vi "Public Application Data Folder.vi"(3 "Relative Path (\"\" - Folder)":string) -> (1 "Client Storage Path":path)   [LabVIEW 2011]
uses:
  <vilib>/Utility/sysdir.llb/System Directory Type.ctl
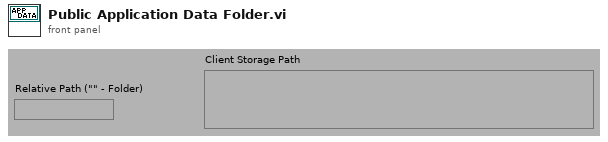
[diagram p1: front panel]
types:
  T1 = enum32{"invalid app kind", "Development System", "Run Time System", "Student Edition", "Embedded LabVIEW", "Evaluation", "Custom"}
  T2 = typedef "System Directory Type.ctl" = i32
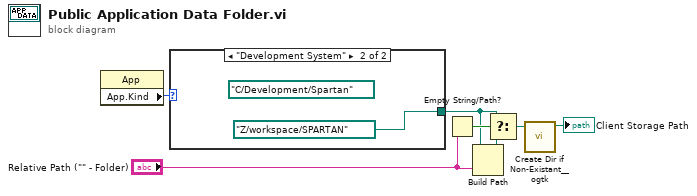
[diagram p0: block diagram]
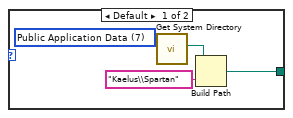
[diagram p2: hidden frame]
diagram:
  n1 = property class="App"() -> ("App.Kind"=w7:T1)  [unwired: 2 in, 2 out]
  n2 = case shown="\"Development System\"" w7 {
    tunnel: [w8 path "Z:/workspace/SPARTAN" ("appended path")] -> w3
    frame Default {
      w10 = T2 7 items=["User Home", "User Desktop", "User Documents", "User Application Data", "User Preferences", "User Temporary", "Public Documents", "Public Application Data", "Public Preferences", "System Core Libraries", "System Installed Libraries", "Application Files", "Boot Volume Root"] ("system directory type")
      n3 = call <vilib>:"Get System Directory.vi"("system directory type"=w10) -> ("system directory"=w9:path)  [unwired: 10 in]
      n4 = Build Path(base path=w9, name or relative path="Kaelus\\Spartan" ("time format string (%c)")) -> (appended path=w8:path)
    }
    frame "Development System" {
      (unwired) path "C:/Development/Spartan" ("appended path")
    }
  }
  n5 = Empty String/Path?(string/path="Relative Path (\"\" - Folder)") -> (empty?=w6:bool)
  n6 = Build Path(base path=w3, name or relative path="Relative Path (\"\" - Folder)") -> (appended path=w5:path)
  n7 = Select(t=w3, s=w6, f=w5) -> (s? t:f=w2:path)
  n8 = call "Create Dir if Non-Existant__ogtk.vi"("Directory Path"=w2) -> ("dup Directory Path"=→"Client Storage Path":path)  [unwired: 2 in, 8 out]
